vi "Post Initialize Action.vi"(8 "error in":errorcluster, 11 "Platform in":refnum<class "Platform.lvclass">) -> (0 "error out":errorcluster, 2 "Init Event Data":variant, 3 "Platform out":refnum<class "Platform.lvclass">)   [LabVIEW 2019, in "Platform.lvlib" / "Platform.lvclass"]
doc: "This VI is called just after the Panel Actor's UI was initialized.\n\nData wired to <b>Init Event Data</b> will be passed in the panel's \"Initialized\" user event.\n\nIf there were any initialization errors they should be handled here.\n\n----\nPlease see the following web address for additional documentation and tutorial information:\nhttp://www.mooregoodideas.com/mgi-panel-manager/\n\nAuthor: Derek Trepanier\n\nCopyright (c) 2018, Moore Good Ideas, Inc.\n\nAll rights reserved.\n\nRedistribution and use in source and binary forms, with or without modification, are permitted provided that the following conditions are met:\n\n * Redistributions of source code must retain the above copyright notice, this list of conditions and the following disclaimer.\n * Redistributions in binary form must reproduce the above copyright notice, this list of conditions and the following disclaimer in the documentation and/or other materials provided with the distribution.\n * Neither the name of Moore Good Ideas, Inc. nor the names of its contributors may be used to endorse or promote products derived from this software without specific prior written permission.\n\nTHIS SOFTWARE IS PROVIDED BY THE COPYRIGHT HOLDERS AND CONTRIBUTORS \"AS IS\" AND ANY EXPRESS OR IMPLIED WARRANTIES, INCLUDING, BUT NOT LIMITED TO, THE IMPLIED WARRANTIES OF MERCHANTABILITY AND FITNESS FOR A PARTICULAR PURPOSE ARE DISCLAIMED. IN NO EVENT SHALL THE COPYRIGHT OWNER OR CONTRIBUTORS BE LIABLE FOR ANY DIRECT, INDIRECT, INCIDENTAL, SPECIAL, EXEMPLARY, OR CONSEQUENTIAL DAMAGES (INCLUDING, BUT NOT LIMITED TO, PROCUREMENT OF SUBSTITUTE GOODS OR SERVICES; LOSS OF USE, DATA, OR PROFITS; OR BUSINESS INTERRUPTION) HOWEVER CAUSED AND ON ANY THEORY OF LIABILITY, WHETHER IN CONTRACT, STRICT LIABILITY, OR TORT (INCLUDING NEGLIGENCE OR OTHERWISE) ARISING IN ANY WAY OUT OF THE USE OF THIS SOFTWARE, EVEN IF ADVISED OF THE POSSIBILITY OF SUCH DAMAGE."
uses:
  Platform.lvclass
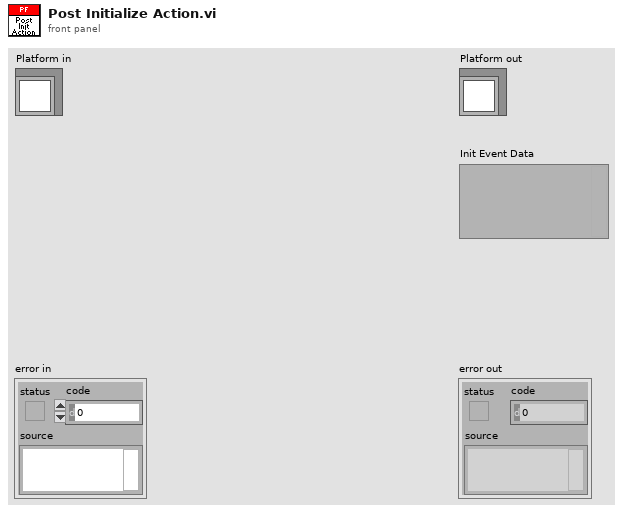
[diagram p1: front panel]
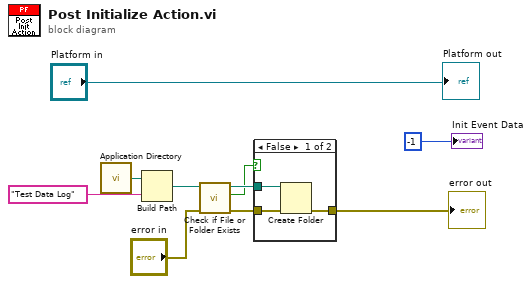
[diagram p0: block diagram]
diagram:
  n1 = call <vilib>:"Application Directory.vi"() -> ("Application Directory"=w5:path)
  n2 = Build Path(base path=w5, name or relative path="Test Data Log" ("relative uri")) -> (appended path=w4:path)
  n3 = call <vilib>:"Check if File or Folder Exists.vi"("error in (no error)"="error in", "path"=w4) -> ("error out"=w8:errorcluster, "file or folder exists?"=w7:bool, "dup path"=w9:path)  [unwired: 7 in]
  n4 = case shown="False" w7 {
    tunnel: w8 -> [w13 w14]
    tunnel: [w12 w14] -> w1
    tunnel: w9 -> [w11 _]
    frame False {
      n5 = Create Folder(path (use dialog)=w11, error in=w13) -> (error out=w12:errorcluster)  [unwired: 1 in, 2 out]
    }
    frame True {
    }
  }
  "error out" <- w1
  "Platform out" <- "Platform in"
  "Init Event Data" <- -1 ("Value (Signaling)")
